vi "Periodic Tasks.vi"(8 "error in":errorcluster) -> ()   [LabVIEW 2018]
doc: "This VI runs in parallel to other tasks. It can contain as many user-defined periodic loops as you need. These can carry out PID or other sorts of timed response."
uses:
  <vilib>/Rock Robotics/WPI/Solenoid/WPI_SolenoidValue.ctl
  <vilib>/Rock Robotics/WPI/ThirdParty/Phoenix-LabVIEW/Motor Controller/Controls/CTRE_Phoenix_MotorControl_ControlMode.ctl
  <vilib>/Rock Robotics/WPI/DriverStation/WPI_DriverStationRobotMode2.ctl
  558dcaf8-7ea7-4920-b857-199f0f95a235.vi
  db2b8676-33c7-4e09-9355-13c98dcb7fd1.vi
  49744297-d732-4f26-b9df-ea13e04ead65.vi
  0c7d2dc5-c582-4743-8fb3-b9c2bdc871ef.vi
  0ab41fdd-f005-4a41-8abb-d0c1aebc8839.vi
  eb1224c5-d191-4a5a-b208-f0176ff8254b.vi
  fa0b2ed9-014b-4d02-a9e7-965de739ed34.vi
  3bc81077-0bee-49a4-9064-f6dc6ff34700.vi
  c6107473-3bbc-4d68-b130-33bb0f28684e.vi
  bc72f310-a025-467b-8a7d-9af20b832017.vi
  627df16c-e363-45ec-ab0c-cc0e3a3b33f7.vi
  9981459b-1b43-4049-8584-415fba4f8944.vi
  f90bc81b-d4ab-4cd4-9451-4feb4d491bc8.vi
  4a955322-911f-44d6-8f01-79f36aab782e.vi
  ea05d6e2-4bc2-4863-96e4-0034388c650a.vi
  93672789-ce46-4bc6-a5b5-faff44e817a8.vi
  c8be7294-c6ee-427e-ae78-3199e8744a18.vi
  1c7609ed-6cb5-470b-bbb9-41d14296924d.vi
  50b6936b-a54e-4087-a151-83919d29fb22.vi
  efed0d96-a490-4904-9cbf-ad4873da1ad9.vi
  96b11e64-b6fc-4637-b85c-b75fecbcb338.vi
  RobotStates.vi
  Robot Global Data.vi
  <vilib>/Rock Robotics/Network Tables/NT Write Number.vi
  RefNums_DriverStation.vi
  <vilib>/Rock Robotics/WPI/Utilities/WPI_GetSetVariantRefNum.vi
  RefNums_Actuators.vi
  <vilib>/Rock Robotics/WPI/Solenoid/WPI_SolenoidSetEnum.vi
  SensorReadings.vi
  Inputs_DriverStation.vi
  RefNums_Sensors.vi
  843581b2-07bb-4a5d-853d-75b7c067592b.vi
  455b4b06-4f38-49e0-865f-ae84c517b9e7.vi
panel:
  out "Sensor Loop (ms)":u32
  in  "Enable Plotting":bool
  out "Control Loop Time (ms)":u32
  out "PID Tracking":cluster{"Goal Wheel Position":dbl, dbl}(graph)={"Goal Wheel Position"=0.0, -90.17571233858979}
  out "Contribution Tracking":cluster{dbl, dbl, dbl}(graph)
  in  "N-Int":i32=50
  in  "N-Diff":i32=50
  in  "Kd":dbl=1e-06
  in  "Ki":dbl=5e-06
  in  "Kp":dbl=3e-05
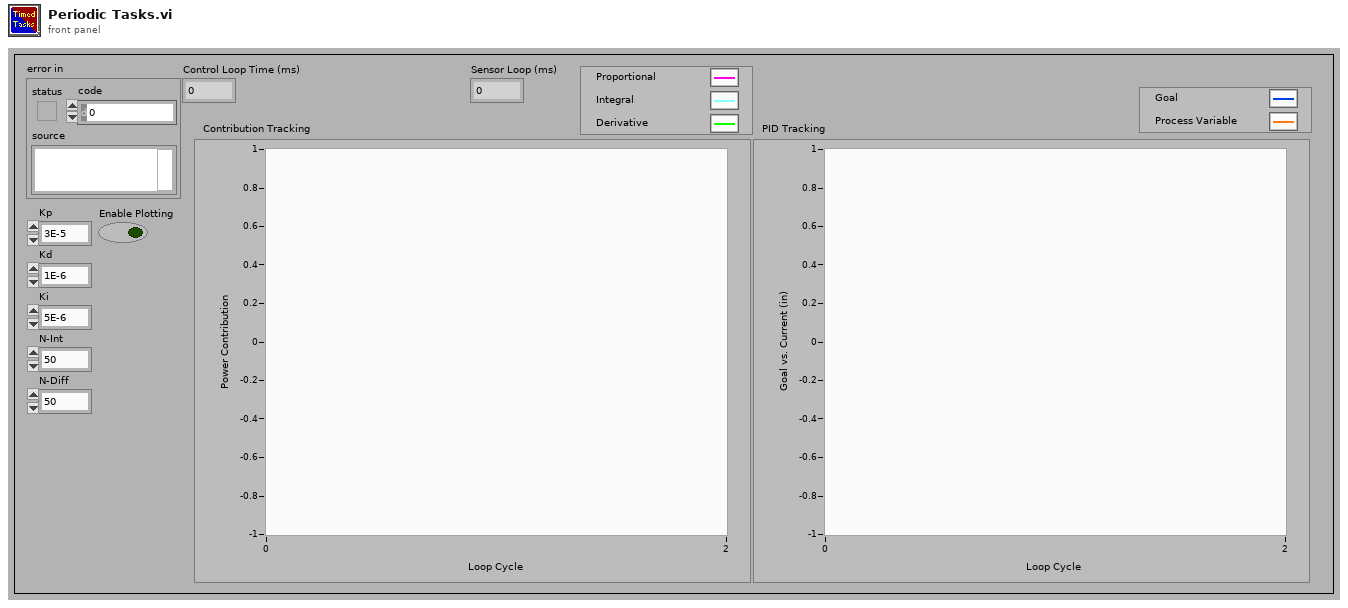
[diagram p1: front panel]
types:
  T1 = typedef "WPI_MotorControlDeviceRef.ctl" = cluster{"DeviceStatus":errorcluster, "Type":T2, "PWM":cluster{"PWM Channel":T3, "DeadBand":T4}, "CAN":cluster{"Device Number":u8, "SetOutput VI Ref":variant, "GetOutput VI Ref":variant, "Enable VI Ref":variant, "Disable VI Ref":variant, "Data":variant}, "Invert":bool, "DIO PWM":cluster{"PWM \"Enable\" Channel":T3, "DIOChannel":T5, "PWM Rate":dbl}}
  T2 = typedef "WPI_MotorControlType.ctl" = enum16{"PWM", "CAN", "DIO PWM"}
  T3 = typedef "FPGA_DIOPWMChannel.ctl" = enum8{"PWM 0", "PWM 1", "PWM 2", "PWM 3", "PWM 4", "PWM 5", "PWM 6", "PWM 7", "PWM 8", "PWM 9", "PWM MXP 0", "PWM MXP 1", "PWM MXP 2", "PWM MXP 3", "PWM MXP 4", "PWM MXP 5", "PWM MXP 6", "PWM MXP 7", "PWM MXP 8", "PWM MXP 9", "Invalid"}
  T4 = typedef "WPI_PWMDeadband.ctl" = cluster{"Name":string, "maxPositivePwm":i32, "minPositivePwm":i32, "centerPwm":i32, "maxNegativePwm":i32, "minNegativePwm":i32, "angularRange":u16}
  T5 = typedef "FPGA_DIOChannel.ctl" = enum8{"DIO 0", "DIO 1", "DIO 2", "DIO 3", "DIO 4", "DIO 5", "DIO 6", "DIO 7", "DIO 8", "DIO 9", "DIO MXP 0", "DIO MXP 1", "DIO MXP 2", "DIO MXP 3", "DIO MXP 4", "DIO MXP 5", "DIO MXP 6", "DIO MXP 7", "DIO MXP 8", "DIO MXP 9", "DIO MXP 10", "DIO MXP 11", "DIO MXP 12", "DIO MXP 13", "DIO MXP 14", "DIO MXP 15", "SPI Port CS1", "SPI Port CS2", "SPI Port CS3", "SPI Port MISO", "SPI Port MOSI", "Invalid"}
  T6 = typedef "WPI_SolenoidDevRef.ctl" = cluster{"DevStatus":errorcluster, "Pneumatics Control Module":u8, "Forward Solenoid Channel":T7, "Reverse Solenoid Channel":T7}
  T7 = typedef "WPI_SolenoidChannel.ctl" = enum8{"Solenoid 0", "Solenoid 1", "Solenoid 2", "Solenoid 3", "Solenoid 4", "Solenoid 5", "Solenoid 6", "Solenoid 7", "Invalid"}
  T8 = typedef "WPI_RobotDriveDevRef.ctl" = cluster{"DevStatus":errorcluster, "Motors[]":T1[], "Square Inputs":bool, "Max Output":dbl}
  T9 = typedef "WPI_JoystickDevRef.ctl" = cluster{"Device":T10}
  T10 = typedef "WPI_JoystickDeviceEnum.ctl" = enum16{"USB 0", "USB 1", "USB 2", "USB 3", "USB 4", "USB 5"}
  T11 = typedef "WPI_CompressorDevRef.ctl" = cluster{"DevStatus":errorcluster, "Pneumatics Control Module":u8}
  T12 = typedef "WPI_AnalogChannelDevRef.ctl" = cluster{"DevStatus":errorcluster, "Analog Channel":T13}
  T13 = typedef "FPGA_AIChannel.ctl" = enum8{"AI 0", "AI 1", "AI 2", "AI 3", "AI MXP 0", "AI MXP 1", "AI MXP 2", "AI MXP 3", "Invalid"}
  T14 = typedef "WPI_DriverStationRobotMode2.ctl" = enum16{"Autonomous Disabled", "Autonomous Enabled", "Teleop Disabled", "Teleop Enabled", "Disconnected", "Finish", "Test Disabled", "Test Enabled", "Emergency Stopped"}
  T15 = typedef "CTRE_Phoenix_MotorControl_ControlMode.ctl" = u16
  T16 = typedef "WPI_SolenoidValue.ctl" = enum16{"Off", "On", "Forward", "Reverse"}
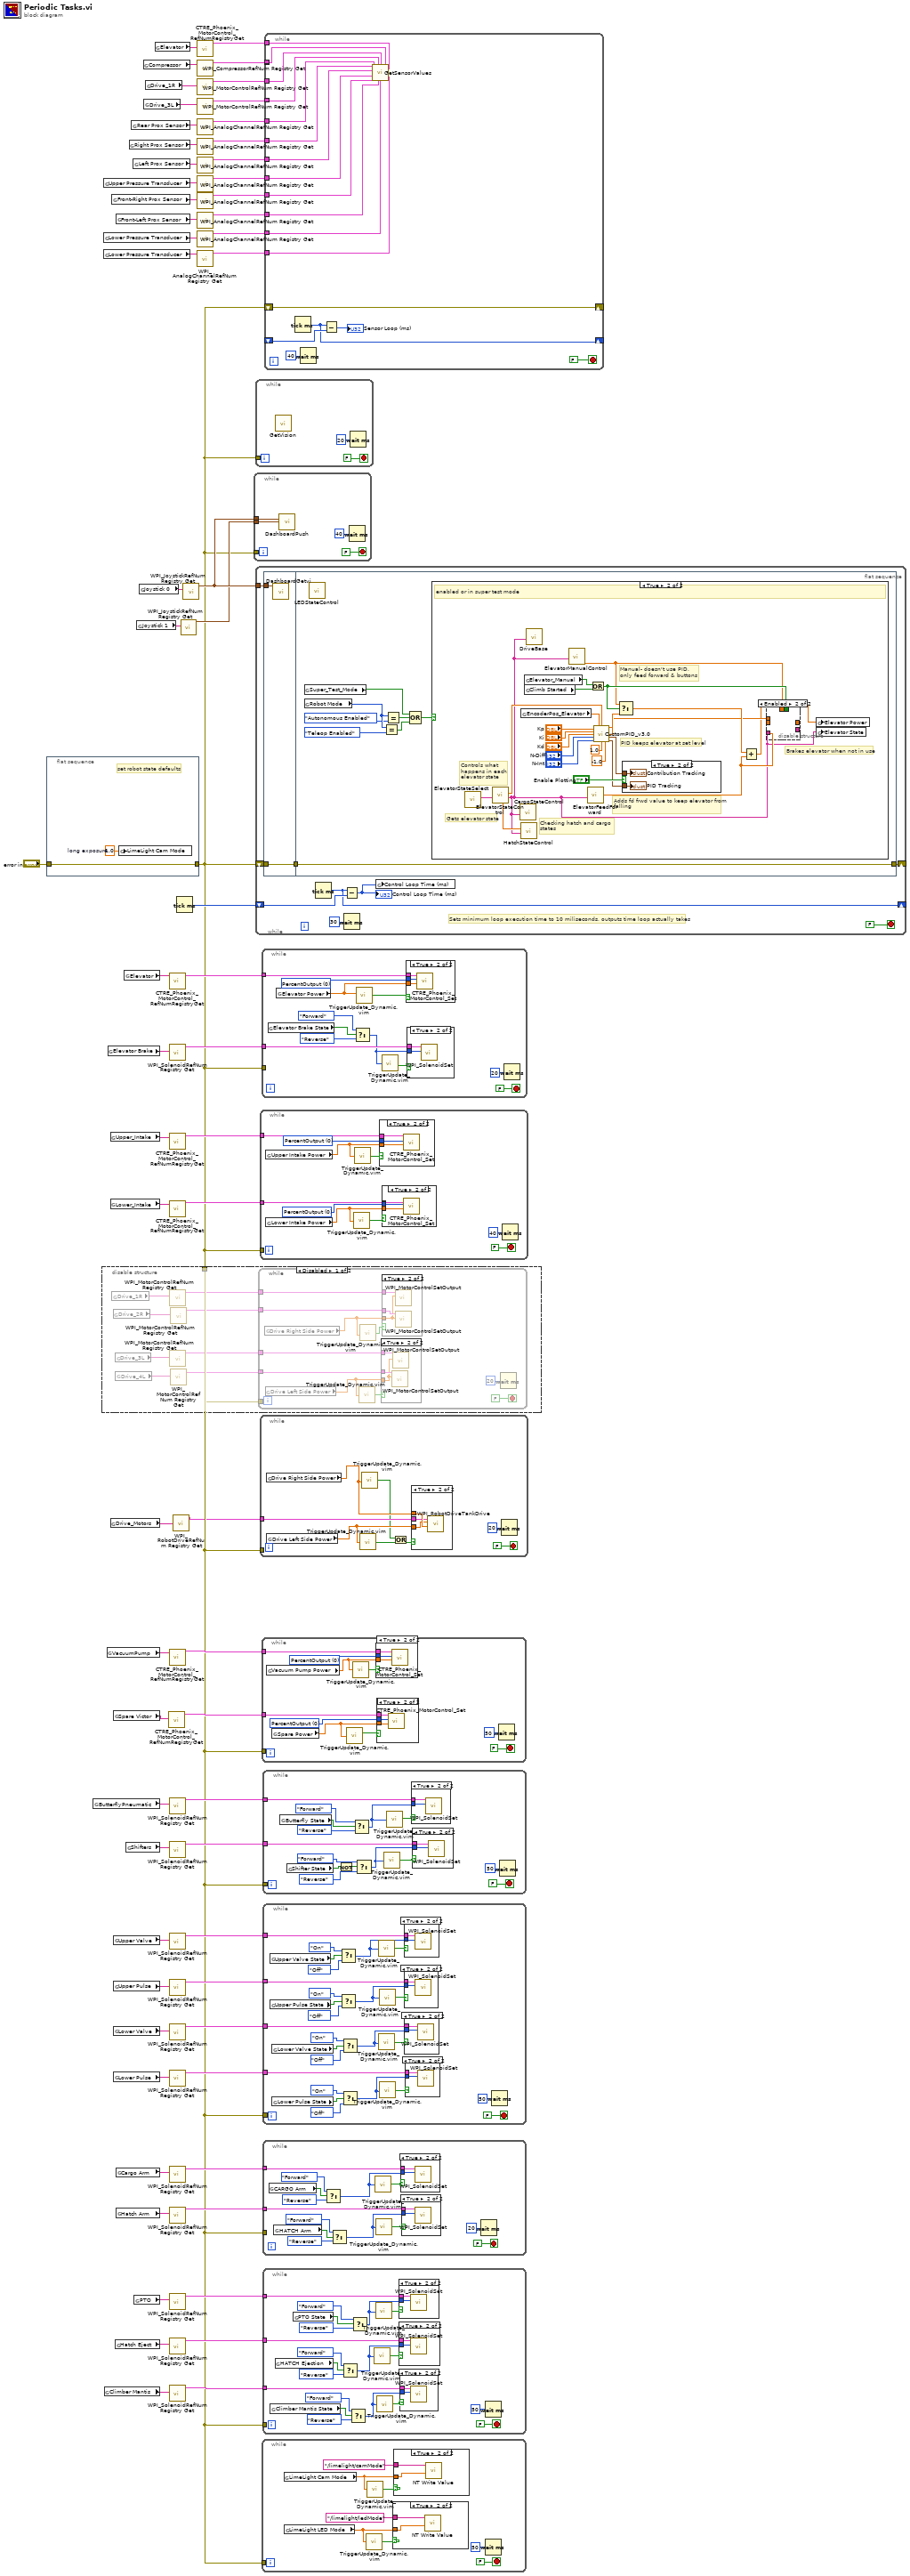
[diagram p0: block diagram]
diagram:
  n1 = flat-sequence {
    tunnel: [w69] -> w3
    tunnel: "error in" -> [w69]
    frame #0 {
      w68 = 1.0  # long exposure
      # "set robot state defaults"
      n2 = global write "RobotStates.vi" "LimeLight Cam Mode"(w68) -> ()
    }
  }
  n3 = global read "RefNums_Actuators.vi" "ButterflyPneumatic"() -> (w65:string)
  n4 = disable-structure shown="Disabled" {
    disable-tunnel: w3 -> [w70 _]
    frame Disabled {
      n5 = global read "RefNums_Actuators.vi" "Drive_1R"() -> (w72:string)
      n6 = global read "RefNums_Actuators.vi" "Drive_2R"() -> (w78:string)
      n7 = global read "RefNums_Actuators.vi" "Drive_3L"() -> (w74:string)
      n8 = global read "RefNums_Actuators.vi" "Drive_4L"() -> (w76:string)
      n9 = call <vilib>:"WPI_MotorControlRefNum Registry Get.vi"("refnum name"=w72) -> ("MotorControlDevRef"=w71:T1)  [unwired: 9 in, 1 out]
      n10 = call <vilib>:"WPI_MotorControlRefNum Registry Get.vi"("refnum name"=w74) -> ("MotorControlDevRef"=w73:T1)  [unwired: 9 in, 1 out]
      n11 = call <vilib>:"WPI_MotorControlRefNum Registry Get.vi"("refnum name"=w76) -> ("MotorControlDevRef"=w75:T1)  [unwired: 9 in, 1 out]
      n12 = call <vilib>:"WPI_MotorControlRefNum Registry Get.vi"("refnum name"=w78) -> ("MotorControlDevRef"=w77:T1)  [unwired: 9 in, 1 out]
      n13 = while {
        tunnel: w77 -> [w88]
        tunnel: w75 -> [w87]
        tunnel: w70 -> [_]
        tunnel: w73 -> [w80]
        tunnel: w71 -> [w79]
        stop <- FALSE stop-if-true
        n14 = global read "RobotStates.vi" "Drive Right Side Power"() -> (w84:dbl)
        n15 = global read "RobotStates.vi" "Drive Left Side Power"() -> (w82:dbl)
        n16 = call "TriggerUpdate_Dynamic.vim"("Trigger"=w82) -> ("Update"=w81:bool)
        n17 = call "TriggerUpdate_Dynamic.vim"("Trigger"=w84) -> ("Update"=w83:bool)
        n18 = case shown="True" w81 {
          tunnel: w87 -> [_ w91]
          tunnel: w82 -> [_ w90]
          tunnel: w80 -> [_ w89]
          frame False {
          }
          frame True {
            n19 = call <vilib>:"WPI_MotorControlSetOutput.vi"("Output"=w90, "MotorControlDevRef"=w91) -> ()  [unwired: 7 in, 3 out]
            n20 = call <vilib>:"WPI_MotorControlSetOutput.vi"("Output"=w90, "MotorControlDevRef"=w89) -> ()  [unwired: 7 in, 3 out]
          }
        }
        n21 = case shown="True" w83 {
          tunnel: w88 -> [_ w94]
          tunnel: w84 -> [_ w93]
          tunnel: w79 -> [_ w92]
          frame False {
          }
          frame True {
            n22 = call <vilib>:"WPI_MotorControlSetOutput.vi"("Output"=w93, "MotorControlDevRef"=w92) -> ()  [unwired: 7 in, 3 out]
            n23 = call <vilib>:"WPI_MotorControlSetOutput.vi"("Output"=w93, "MotorControlDevRef"=w94) -> ()  [unwired: 7 in, 3 out]
          }
        }
        n24 = Wait (ms)(milliseconds to wait=u32 20) -> ()  [unwired: 1 out]
      }
    }
    frame Enabled {
    }
  }
  n25 = global read "RefNums_Sensors.vi" "Upper Pressure Transducer"() -> (w23:string)
  n26 = global read "RefNums_Sensors.vi" "Lower Pressure Transducer"() -> (w22:string)
  n27 = global read "RefNums_Sensors.vi" "Lower Pressure Transducer"() -> (w19:string)
  n28 = global read "RefNums_Actuators.vi" "Climber Mantis"() -> (w44:string)
  n29 = global read "RefNums_Actuators.vi" "VacuumPump"() -> (w58:string)
  n30 = global read "RefNums_Actuators.vi" "Elevator Brake"() -> (w47:string)
  n31 = global read "RefNums_Actuators.vi" "Upper_Intake"() -> (w55:string)
  n32 = global read "RefNums_Actuators.vi" "Lower_Intake"() -> (w54:string)
  n33 = global read "RefNums_Actuators.vi" "Drive_Motors"() -> (w2:string)
  n34 = global read "RefNums_Sensors.vi" "Front-Right Prox Sensor"() -> (w20:string)
  n35 = global read "RefNums_Actuators.vi" "Spare Victor"() -> (w51:string)
  n36 = global read "RefNums_Actuators.vi" "Upper Valve"() -> (w40:string)
  n37 = global read "RefNums_Actuators.vi" "Upper Pulse"() -> (w61:string)
  n38 = global read "RefNums_Actuators.vi" "Lower Valve"() -> (w38:string)
  n39 = global read "RefNums_Actuators.vi" "Lower Pulse"() -> (w36:string)
  n40 = global read "RefNums_Actuators.vi" "Hatch Eject"() -> (w45:string)
  n41 = global read "RefNums_Sensors.vi" "Front-Left Prox Sensor"() -> (w21:string)
  n42 = global read "RefNums_Actuators.vi" "Cargo Arm"() -> (w57:string)
  n43 = global read "RefNums_Actuators.vi" "Hatch Arm"() -> (w46:string)
  n44 = global read "RefNums_Actuators.vi" "Elevator"() -> (w11:string)
  n45 = global read "RefNums_Actuators.vi" "Shifters"() -> (w63:string)
  n46 = global read "RefNums_Sensors.vi" "Right Prox Sensor"() -> (w27:string)
  n47 = global read "RefNums_Sensors.vi" "Rear Prox Sensor"() -> (w29:string)
  n48 = global read "RefNums_Sensors.vi" "Left Prox Sensor"() -> (w28:string)
  n49 = global read "RefNums_Actuators.vi" "PTO"() -> (w49:string)
  n50 = global read "RefNums_DriverStation.vi" "Joystick 1"() -> (w10:string)
  n51 = global read "RefNums_DriverStation.vi" "Joystick 0"() -> (w66:string)
  n52 = global read "RefNums_Actuators.vi" "Compressor"() -> (w33:string)
  n53 = global read "RefNums_Actuators.vi" "Drive_3L"() -> (w6:string)
  n54 = global read "RefNums_Actuators.vi" "Drive_1R"() -> (w7:string)
  n55 = global read "RefNums_Actuators.vi" "Elevator"() -> (w32:string)
  n56 = call <vilib>:"CTRE_Phoenix_MotorControl_RefNumRegistryGet.vi"("refnum name"=w51) -> ("PhoenixMotorControlDevRef"=w50:T1)  [unwired: 9 in, 1 out]
  n57 = call <vilib>:"CTRE_Phoenix_MotorControl_RefNumRegistryGet.vi"("refnum name"=w11) -> ("PhoenixMotorControlDevRef"=w67:T1)  [unwired: 9 in, 1 out]
  n58 = call <vilib>:"WPI_SolenoidRefNum Registry Get.vi"("refnum name"=w47) -> ("SolenoidDevRef"=w13:T6)  [unwired: 9 in, 1 out]
  n59 = call <vilib>:"CTRE_Phoenix_MotorControl_RefNumRegistryGet.vi"("refnum name"=w55) -> ("PhoenixMotorControlDevRef"=w53:T1)  [unwired: 9 in, 1 out]
  n60 = call <vilib>:"CTRE_Phoenix_MotorControl_RefNumRegistryGet.vi"("refnum name"=w54) -> ("PhoenixMotorControlDevRef"=w52:T1)  [unwired: 9 in, 1 out]
  n61 = call <vilib>:"CTRE_Phoenix_MotorControl_RefNumRegistryGet.vi"("refnum name"=w58) -> ("PhoenixMotorControlDevRef"=w59:T1)  [unwired: 9 in, 1 out]
  n62 = call <vilib>:"WPI_SolenoidRefNum Registry Get.vi"("refnum name"=w65) -> ("SolenoidDevRef"=w64:T6)  [unwired: 9 in, 1 out]
  n63 = call <vilib>:"WPI_SolenoidRefNum Registry Get.vi"("refnum name"=w63) -> ("SolenoidDevRef"=w62:T6)  [unwired: 9 in, 1 out]
  n64 = call <vilib>:"WPI_SolenoidRefNum Registry Get.vi"("refnum name"=w40) -> ("SolenoidDevRef"=w39:T6)  [unwired: 9 in, 1 out]
  n65 = call <vilib>:"WPI_SolenoidRefNum Registry Get.vi"("refnum name"=w61) -> ("SolenoidDevRef"=w60:T6)  [unwired: 9 in, 1 out]
  n66 = call <vilib>:"WPI_SolenoidRefNum Registry Get.vi"("refnum name"=w38) -> ("SolenoidDevRef"=w37:T6)  [unwired: 9 in, 1 out]
  n67 = call <vilib>:"WPI_SolenoidRefNum Registry Get.vi"("refnum name"=w36) -> ("SolenoidDevRef"=w35:T6)  [unwired: 9 in, 1 out]
  n68 = call <vilib>:"WPI_SolenoidRefNum Registry Get.vi"("refnum name"=w57) -> ("SolenoidDevRef"=w56:T6)  [unwired: 9 in, 1 out]
  n69 = call <vilib>:"WPI_SolenoidRefNum Registry Get.vi"("refnum name"=w46) -> ("SolenoidDevRef"=w43:T6)  [unwired: 9 in, 1 out]
  n70 = call <vilib>:"WPI_SolenoidRefNum Registry Get.vi"("refnum name"=w49) -> ("SolenoidDevRef"=w48:T6)  [unwired: 9 in, 1 out]
  n71 = call <vilib>:"WPI_SolenoidRefNum Registry Get.vi"("refnum name"=w45) -> ("SolenoidDevRef"=w42:T6)  [unwired: 9 in, 1 out]
  n72 = call <vilib>:"WPI_SolenoidRefNum Registry Get.vi"("refnum name"=w44) -> ("SolenoidDevRef"=w41:T6)  [unwired: 9 in, 1 out]
  n73 = call <vilib>:"WPI_RobotDriveRefNum Registry Get.vi"("refnum name"=w2) -> ("RobotDriveDevRef"=w1:T8)  [unwired: 9 in, 1 out]
  n74 = Tick Count (ms)() -> (millisecond timer value=w34:u32)
  n75 = call <vilib>:"WPI_JoystickRefNum Registry Get.vi"("refnum name"=w10) -> ("JoystickDevRef"=w9:T9)  [unwired: 9 in, 1 out]
  n76 = call <vilib>:"WPI_JoystickRefNum Registry Get.vi"("refnum name"=w66) -> ("JoystickDevRef"=w12:T9)  [unwired: 9 in, 1 out]
  n77 = call <vilib>:"CTRE_Phoenix_MotorControl_RefNumRegistryGet.vi"("refnum name"=w32) -> ("PhoenixMotorControlDevRef"=w31:T1)  [unwired: 9 in, 1 out]
  n78 = call <vilib>:"WPI_CompressorRefNum Registry Get.vi"("refnum name"=w33) -> ("CompressorDevRef"=w30:T11)  [unwired: 9 in, 1 out]
  n79 = call <vilib>:"WPI_MotorControlRefNum Registry Get.vi"("refnum name"=w7) -> ("MotorControlDevRef"=w5:T1)  [unwired: 9 in, 1 out]
  n80 = call <vilib>:"WPI_MotorControlRefNum Registry Get.vi"("refnum name"=w6) -> ("MotorControlDevRef"=w4:T1)  [unwired: 9 in, 1 out]
  n81 = call <vilib>:"WPI_AnalogChannelRefNum Registry Get.vi"("refnum name"=w29) -> ("AIDeviceRef"=w26:T12)  [unwired: 9 in, 1 out]
  n82 = call <vilib>:"WPI_AnalogChannelRefNum Registry Get.vi"("refnum name"=w27) -> ("AIDeviceRef"=w25:T12)  [unwired: 9 in, 1 out]
  n83 = call <vilib>:"WPI_AnalogChannelRefNum Registry Get.vi"("refnum name"=w28) -> ("AIDeviceRef"=w24:T12)  [unwired: 9 in, 1 out]
  n84 = call <vilib>:"WPI_AnalogChannelRefNum Registry Get.vi"("refnum name"=w23) -> ("AIDeviceRef"=w18:T12)  [unwired: 9 in, 1 out]
  n85 = call <vilib>:"WPI_AnalogChannelRefNum Registry Get.vi"("refnum name"=w20) -> ("AIDeviceRef"=w17:T12)  [unwired: 9 in, 1 out]
  n86 = call <vilib>:"WPI_AnalogChannelRefNum Registry Get.vi"("refnum name"=w21) -> ("AIDeviceRef"=w16:T12)  [unwired: 9 in, 1 out]
  n87 = call <vilib>:"WPI_AnalogChannelRefNum Registry Get.vi"("refnum name"=w22) -> ("AIDeviceRef"=w15:T12)  [unwired: 9 in, 1 out]
  n88 = call <vilib>:"WPI_AnalogChannelRefNum Registry Get.vi"("refnum name"=w19) -> ("AIDeviceRef"=w14:T12)  [unwired: 9 in, 1 out]
  n89 = while {
    tunnel: w12 -> [w97]
    tunnel: w3 -> [_]
    tunnel: w9 -> [w95]
    stop <- FALSE stop-if-true
    n90 = call "DashboardPush.vi"("Joystick 0 Ref"=w97, "Joystick 1 Ref"=w95) -> ()  [unwired: 14 in]
    n91 = Wait (ms)(milliseconds to wait=u32 40) -> ()  [unwired: 1 out]
  }
  n92 = while {
    tunnel: w3 -> [_]
    stop <- FALSE stop-if-true
    n93 = call "GetVision.vi"() -> ()  [unwired: 12 in]
    n94 = Wait (ms)(milliseconds to wait=u32 20) -> ()  [unwired: 1 out]
  }
  n95 = while {
    shift-right: [w105] -> _
    shift-left: w3 -> [w107]
    tunnel: w12 -> [w104]
    shift-right: [w102] -> _
    shift-left: w34 -> [w103]
    stop <- FALSE stop-if-true
    # "Sets minimum loop execution time to 10 miliseconds, outputs time loop actually takes"
    n96 = flat-sequence {
      tunnel: w104 -> [w111]
      tunnel: w107 -> [w110]
      tunnel: [w110] -> w106
      tunnel: w106 -> [w119]
      tunnel: [w119] -> w105
      frame #0 {
        n97 = call "DashboardGetvi.vi"("Joystick 1"=w111) -> ()  [unwired: 9 in]
      }
      frame #1 {
        n98 = global read "Inputs_DriverStation.vi" "Super_Test_Mode"() -> (w112:bool)
        n99 = global read "Robot Global Data.vi" "Robot Mode"() -> (w116:T14)
        n100 = call "LEDStateControl.vi"() -> ()  [unwired: 12 in]
        n101 = Equal?(x=w116, y=WPI_DriverStationRobotMode2."Teleop Enabled") -> (x = y?=w117:bool)
        n102 = Equal?(x=w116, y=WPI_DriverStationRobotMode2."Autonomous Enabled") -> (x = y?=w118:bool)
        n103 = Compound Arithmetic op=OR(w112, w118, w117) -> (w113:bool)
        n104 = case shown="True" w113 {
          frame False {
            # "disabled and not in super test mode"
          }
          frame True {
            # "Brakes elevator when not in use"
            # "PID keeps elevator at set level"
            # "Manual- doesn't use PID,\nonly feed forward & buttons"
            # "Adds fd frwd value to keep elevator from falling"
            # "Checking hatch and cargo \nstates"
            # "Controls what\nhappens in each \nelevator state"
            # "Gets elevator state"
            # "enabled or in super test mode"
            n105 = call "ElevatorStateSelect.vi"() -> ("Elevator State"=w140:string)  [unwired: 11 in]
            n106 = call "ElevatorStateControl.vi"("Elevator State"=w140) -> ("Elevator State Out"=w121:string, "Target Elevator Position"=w138:dbl, "Target Vacuum Pump Power"=w127:dbl)  [unwired: 8 in]
            n107 = call "CargoStateControl.vi"("Elevator State"=w121) -> ()  [unwired: 11 in]
            n108 = call "HatchStateControl.vi"("Elevator State"=w121, "Vacuum Pump Power"=w127) -> ()  [unwired: 10 in]
            n109 = global read "SensorReadings.vi" "EncoderPos_Elevator"() -> (w137:dbl)
            n110 = global read "Inputs_DriverStation.vi" "Elevator_Manual"() -> (w123:bool)
            n111 = global read "RobotStates.vi" "Climb Started"() -> (w122:bool)
            n112 = call "DriveBase.vi"("Elevator State"=w121) -> ()  [unwired: 11 in]
            n113 = call "ElevatorManualControl.vi"("Elevator State"=w121) -> ("Manual Contribution"=w126:dbl)  [unwired: 10 in]
            n114 = call "ElevatorFeedForward.vi"("Elevator State"=w121) -> ("Feed Forward Contribution"=w124:dbl)  [unwired: 10 in]
            n115 = Or(x=w123, y=w122) -> (x .or. y?=w143:bool)
            n116 = call "CustomPID_v3.0.vi"("Kp"="Kp", "Process Variable"=w137, "Goal"=w138, "Ki"="Ki", "Kd"="Kd", "N-Diff"="N-Diff", "N-Int"="N-Int", "Max Ouput"=1.0, "Min Output"=-1.0) -> ("Current Error"=w125:dbl, "Command"=w139:dbl, "Contribution Tracking"=w129:cluster{dbl, dbl, dbl}, "PID Tracking"=w128:cluster{"Goal Wheel Position":dbl, dbl})  [unwired: 3 in]
            n117 = Select(t=w126, s=w143, f=w139) -> (s? t:f=w141:dbl)
            n118 = case shown="True" "Enable Plotting" {
              tunnel: w129 -> [_ w153]
              tunnel: w128 -> [_ w152]
              frame False {
              }
              frame True {
                "Contribution Tracking" <- w153
                "PID Tracking" <- w152
              }
            }
            n119 = Add(x=w141, y=w124) -> (x+y=w120:dbl)
            n120 = disable-structure shown="Enabled" {
              disable-tunnel: w143 -> [w151 _]
              disable-tunnel: _ -> [w150 _]
              disable-tunnel: [w149 _] -> _
              disable-tunnel: [w148 _] -> _
              disable-tunnel: w126 -> [w147 _]
              disable-tunnel: w125 -> [w146 _]
              disable-tunnel: w124 -> [w145 _]
              disable-tunnel: w121 -> [w144 _]
              frame Disabled {
                n121 = call "ElevatorBrake.vi"("Elevator Manual Mode"=w151, "Manual Movement"=w147, "Feed Forward Contribution"=w145, "Elevator State In"=w144, "Elevator Power In"=w150, "Elevator Error"=w146) -> ("Elevator State Out"=w148:string, "Elevator Power Out"=w149:dbl)  [unwired: 4 in]
              }
              frame Enabled {
              }
            }
            n122 = global write "RobotStates.vi" "Elevator Power"(w120) -> ()
            n123 = global write "RobotStates.vi" "Elevator State"(w121) -> ()
          }
        }
      }
    }
    n124 = Tick Count (ms)() -> (millisecond timer value=w102:u32)
    n125 = Wait (ms)(milliseconds to wait=u32 30) -> ()  [unwired: 1 out]
    n126 = Subtract(x=w102, y=w103) -> (x-y=w101:u32)
    "Control Loop Time (ms)" <- w101
    n127 = global write "SensorReadings.vi" "Control Loop Time (ms)"(w101) -> ()
  }
  n128 = while {
    tunnel: w53 -> [w163]
    tunnel: w52 -> [w162]
    tunnel: w3 -> [_]
    stop <- FALSE stop-if-true
    w160 = T15 0 items=["PercentOutput"=0, "Position"=1, "Velocity"=2, "Current"=3, "Follower"=5, "MotionProfile"=6, "MotionMagic"=7, "MotionProfileArc"=10, "Disabled"=15] ("Control Mode")
    w161 = T15 0 items=["PercentOutput"=0, "Position"=1, "Velocity"=2, "Current"=3, "Follower"=5, "MotionProfile"=6, "MotionMagic"=7, "MotionProfileArc"=10, "Disabled"=15] ("Control Mode")
    n129 = global read "RobotStates.vi" "Upper Intake Power"() -> (w157:dbl)
    n130 = global read "RobotStates.vi" "Lower Intake Power"() -> (w155:dbl)
    n131 = call "TriggerUpdate_Dynamic.vim"("Trigger"=w155) -> ("Update"=w154:bool)
    n132 = call "TriggerUpdate_Dynamic.vim"("Trigger"=w157) -> ("Update"=w156:bool)
    n133 = case shown="True" w156 {
      tunnel: w163 -> [_ w169]
      tunnel: w161 -> [_ w168]
      tunnel: w157 -> [_ w167]
      frame False {
      }
      frame True {
        n134 = call <vilib>:"CTRE_Phoenix_MotorControl_Set.vi"("Output"=w167, "Control Mode"=w168, "PhoenixMotorControlDevRef"=w169) -> ()  [unwired: 7 in, 2 out]
      }
    }
    n135 = case shown="True" w154 {
      tunnel: w162 -> [_ w166]
      tunnel: w160 -> [_ w165]
      tunnel: w155 -> [_ w164]
      frame False {
      }
      frame True {
        n136 = call <vilib>:"CTRE_Phoenix_MotorControl_Set.vi"("Output"=w164, "Control Mode"=w165, "PhoenixMotorControlDevRef"=w166) -> ()  [unwired: 7 in, 2 out]
      }
    }
    n137 = Wait (ms)(milliseconds to wait=u32 40) -> ()  [unwired: 1 out]
  }
  n138 = while {
    tunnel: w1 -> [w177]
    tunnel: w3 -> [_]
    stop <- FALSE stop-if-true
    n139 = global read "RobotStates.vi" "Drive Right Side Power"() -> (w172:dbl)
    n140 = global read "RobotStates.vi" "Drive Left Side Power"() -> (w174:dbl)
    n141 = call "TriggerUpdate_Dynamic.vim"("Trigger"=w174) -> ("Update"=w173:bool)
    n142 = call "TriggerUpdate_Dynamic.vim"("Trigger"=w172) -> ("Update"=w170:bool)
    n143 = Or(x=w170, y=w173) -> (x .or. y?=w171:bool)
    n144 = case shown="True" w171 {
      tunnel: w177 -> [_ w178]
      tunnel: w174 -> [_ w179]
      tunnel: w172 -> [_ w180]
      frame False {
      }
      frame True {
        n145 = call <vilib>:"WPI_RobotDriveTankDrive.vi"("Right axis value"=w180, "Left axis value"=w179, "RobotDriveDevRef"=w178) -> ()  [unwired: 6 in, 3 out]
      }
    }
    n146 = Wait (ms)(milliseconds to wait=u32 20) -> ()  [unwired: 1 out]
  }
  n147 = while {
    tunnel: w3 -> [_]
    tunnel: w13 -> [w187]
    tunnel: w67 -> [w186]
    stop <- FALSE stop-if-true
    w185 = T15 0 items=["PercentOutput"=0, "Position"=1, "Velocity"=2, "Current"=3, "Follower"=5, "MotionProfile"=6, "MotionMagic"=7, "MotionProfileArc"=10, "Disabled"=15] ("Control Mode")
    n148 = global read "RobotStates.vi" "Elevator Brake State"() -> (w190:bool)
    n149 = global read "RobotStates.vi" "Elevator Power"() -> (w184:dbl)
    n150 = Select(t=WPI_SolenoidValue."Forward" ("Value"), s=w190, f=WPI_SolenoidValue."Reverse") -> (s? t:f=w182:T16)
    n151 = call "TriggerUpdate_Dynamic.vim"("Trigger"=w184) -> ("Update"=w183:bool)
    n152 = call "TriggerUpdate_Dynamic.vim"("Trigger"=w182) -> ("Update"=w181:bool)
    n153 = case shown="True" w183 {
      tunnel: w186 -> [_ w195]
      tunnel: w185 -> [_ w194]
      tunnel: w184 -> [_ w193]
      frame False {
      }
      frame True {
        n154 = call <vilib>:"CTRE_Phoenix_MotorControl_Set.vi"("Output"=w193, "Control Mode"=w194, "PhoenixMotorControlDevRef"=w195) -> ()  [unwired: 7 in, 2 out]
      }
    }
    n155 = case shown="True" w181 {
      tunnel: w187 -> [_ w197]
      tunnel: w182 -> [_ w196]
      frame False {
      }
      frame True {
        n156 = call-poly <vilib>:"WPI_SolenoidSet.vi"("Value"=w196, "SolenoidDevRef"=w197) -> ()  [unwired: 8 in, 2 out]
      }
    }
    n157 = Wait (ms)(milliseconds to wait=u32 20) -> ()  [unwired: 1 out]
  }
  n158 = while {
    tunnel: w59 -> [w207]
    tunnel: w50 -> [w206]
    tunnel: w3 -> [_]
    stop <- FALSE stop-if-true
    w198 = T15 0 items=["PercentOutput"=0, "Position"=1, "Velocity"=2, "Current"=3, "Follower"=5, "MotionProfile"=6, "MotionMagic"=7, "MotionProfileArc"=10, "Disabled"=15] ("Control Mode")
    w205 = T15 0 items=["PercentOutput"=0, "Position"=1, "Velocity"=2, "Current"=3, "Follower"=5, "MotionProfile"=6, "MotionMagic"=7, "MotionProfileArc"=10, "Disabled"=15] ("Control Mode")
    n159 = global read "RobotStates.vi" "Vacuum Pump Power"() -> (w202:dbl)
    n160 = global read "RobotStates.vi" "Spare Power"() -> (w200:dbl)
    n161 = call "TriggerUpdate_Dynamic.vim"("Trigger"=w200) -> ("Update"=w199:bool)
    n162 = call "TriggerUpdate_Dynamic.vim"("Trigger"=w202) -> ("Update"=w201:bool)
    n163 = case shown="True" w201 {
      tunnel: w207 -> [_ w213]
      tunnel: w205 -> [_ w212]
      tunnel: w202 -> [_ w211]
      frame False {
      }
      frame True {
        n164 = call <vilib>:"CTRE_Phoenix_MotorControl_Set.vi"("Output"=w211, "Control Mode"=w212, "PhoenixMotorControlDevRef"=w213) -> ()  [unwired: 7 in, 2 out]
      }
    }
    n165 = case shown="True" w199 {
      tunnel: w206 -> [_ w210]
      tunnel: w198 -> [_ w209]
      tunnel: w200 -> [_ w208]
      frame False {
      }
      frame True {
        n166 = call <vilib>:"CTRE_Phoenix_MotorControl_Set.vi"("Output"=w208, "Control Mode"=w209, "PhoenixMotorControlDevRef"=w210) -> ()  [unwired: 7 in, 2 out]
      }
    }
    n167 = Wait (ms)(milliseconds to wait=u32 50) -> ()  [unwired: 1 out]
  }
  n168 = while {
    tunnel: w3 -> [_]
    stop <- FALSE stop-if-true
    n169 = global read "RobotStates.vi" "LimeLight Cam Mode"() -> (w214:dbl)
    n170 = global read "RobotStates.vi" "LimeLight LED Mode"() -> (w217:dbl)
    n171 = call "TriggerUpdate_Dynamic.vim"("Trigger"=w217) -> ("Update"=w219:bool)
    n172 = call "TriggerUpdate_Dynamic.vim"("Trigger"=w214) -> ("Update"=w216:bool)
    n173 = case shown="True" w219 {
      tunnel: "/limelight/ledMode" ("Name") -> [_ w225]
      tunnel: w217 -> [_ w224]
      frame False {
      }
      frame True {
        n174 = call-poly <vilib>:"NT Write Value.vi"("Numeric"=w224, "Name"=w225) -> ()  [unwired: 9 in, 1 out]
      }
    }
    n175 = case shown="True" w216 {
      tunnel: "/limelight/camMode" ("Name") -> [_ w223]
      tunnel: w214 -> [_ w222]
      frame False {
      }
      frame True {
        n176 = call-poly <vilib>:"NT Write Value.vi"("Numeric"=w222, "Name"=w223) -> ()  [unwired: 9 in, 1 out]
      }
    }
    n177 = Wait (ms)(milliseconds to wait=u32 50) -> ()  [unwired: 1 out]
  }
  n178 = while {
    tunnel: w56 -> [w239]
    tunnel: w43 -> [w238]
    tunnel: w3 -> [_]
    stop <- FALSE stop-if-true
    n179 = global read "RobotStates.vi" "CARGO Arm"() -> (w237:bool)
    n180 = global read "RobotStates.vi" "HATCH Arm"() -> (w234:bool)
    n181 = Select(t=WPI_SolenoidValue."Forward" ("Value"), s=w237, f=WPI_SolenoidValue."Reverse") -> (s? t:f=w229:T16)
    n182 = Select(t=WPI_SolenoidValue."Forward" ("Value"), s=w234, f=WPI_SolenoidValue."Reverse") -> (s? t:f=w227:T16)
    n183 = call "TriggerUpdate_Dynamic.vim"("Trigger"=w229) -> ("Update"=w228:bool)
    n184 = call "TriggerUpdate_Dynamic.vim"("Trigger"=w227) -> ("Update"=w226:bool)
    n185 = case shown="True" w228 {
      tunnel: w239 -> [_ w243]
      tunnel: w229 -> [_ w242]
      frame False {
      }
      frame True {
        n186 = call-poly <vilib>:"WPI_SolenoidSet.vi"("Value"=w242, "SolenoidDevRef"=w243) -> ()  [unwired: 8 in, 2 out]
      }
    }
    n187 = case shown="True" w226 {
      tunnel: w238 -> [_ w241]
      tunnel: w227 -> [_ w240]
      frame False {
      }
      frame True {
        n188 = call-poly <vilib>:"WPI_SolenoidSet.vi"("Value"=w240, "SolenoidDevRef"=w241) -> ()  [unwired: 8 in, 2 out]
      }
    }
    n189 = Wait (ms)(milliseconds to wait=u32 20) -> ()  [unwired: 1 out]
  }
  n190 = while {
    tunnel: w48 -> [w263]
    tunnel: w42 -> [w262]
    tunnel: w41 -> [w261]
    tunnel: w3 -> [_]
    stop <- FALSE stop-if-true
    n191 = global read "RobotStates.vi" "Climber Mantis State"() -> (w256:bool)
    n192 = global read "RobotStates.vi" "HATCH Ejection"() -> (w258:bool)
    n193 = global read "RobotStates.vi" "PTO State"() -> (w244:bool)
    n194 = Select(t=WPI_SolenoidValue."Forward" ("Value"), s=w258, f=WPI_SolenoidValue."Reverse") -> (s? t:f=w248:T16)
    n195 = Select(t=WPI_SolenoidValue."Forward" ("Value"), s=w256, f=WPI_SolenoidValue."Reverse") -> (s? t:f=w246:T16)
    n196 = Select(t=WPI_SolenoidValue."Forward" ("Value"), s=w244, f=WPI_SolenoidValue."Reverse") -> (s? t:f=w250:T16)
    n197 = call "TriggerUpdate_Dynamic.vim"("Trigger"=w248) -> ("Update"=w247:bool)
    n198 = call "TriggerUpdate_Dynamic.vim"("Trigger"=w250) -> ("Update"=w249:bool)
    n199 = call "TriggerUpdate_Dynamic.vim"("Trigger"=w246) -> ("Update"=w245:bool)
    n200 = case shown="True" w249 {
      tunnel: w263 -> [_ w269]
      tunnel: w250 -> [_ w268]
      frame False {
      }
      frame True {
        n201 = call-poly <vilib>:"WPI_SolenoidSet.vi"("Value"=w268, "SolenoidDevRef"=w269) -> ()  [unwired: 8 in, 2 out]
      }
    }
    n202 = case shown="True" w247 {
      tunnel: w262 -> [_ w267]
      tunnel: w248 -> [_ w266]
      frame False {
      }
      frame True {
        n203 = call-poly <vilib>:"WPI_SolenoidSet.vi"("Value"=w266, "SolenoidDevRef"=w267) -> ()  [unwired: 8 in, 2 out]
      }
    }
    n204 = case shown="True" w245 {
      tunnel: w261 -> [_ w265]
      tunnel: w246 -> [_ w264]
      frame False {
      }
      frame True {
        n205 = call-poly <vilib>:"WPI_SolenoidSet.vi"("Value"=w264, "SolenoidDevRef"=w265) -> ()  [unwired: 8 in, 2 out]
      }
    }
    n206 = Wait (ms)(milliseconds to wait=u32 50) -> ()  [unwired: 1 out]
  }
  n207 = while {
    tunnel: w64 -> [w284]
    tunnel: w62 -> [w283]
    tunnel: w3 -> [_]
    stop <- FALSE stop-if-true
    n208 = global read "RobotStates.vi" "Butterfly State"() -> (w280:bool)
    n209 = global read "RobotStates.vi" "Shifter State"() -> (w279:bool)
    n210 = Not(x=w279) -> (.not. x?=w270:bool)
    n211 = Select(t=WPI_SolenoidValue."Forward" ("Value"), s=w280, f=WPI_SolenoidValue."Reverse") -> (s? t:f=w274:T16)
    n212 = Select(t=WPI_SolenoidValue."Forward" ("Value"), s=w270, f=WPI_SolenoidValue."Reverse") -> (s? t:f=w272:T16)
    n213 = call "TriggerUpdate_Dynamic.vim"("Trigger"=w272) -> ("Update"=w271:bool)
    n214 = call "TriggerUpdate_Dynamic.vim"("Trigger"=w274) -> ("Update"=w273:bool)
    n215 = case shown="True" w273 {
      tunnel: w284 -> [_ w288]
      tunnel: w274 -> [_ w287]
      frame False {
      }
      frame True {
        n216 = call-poly <vilib>:"WPI_SolenoidSet.vi"("Value"=w287, "SolenoidDevRef"=w288) -> ()  [unwired: 8 in, 2 out]
      }
    }
    n217 = case shown="True" w271 {
      tunnel: w283 -> [_ w286]
      tunnel: w272 -> [_ w285]
      frame False {
      }
      frame True {
        n218 = call-poly <vilib>:"WPI_SolenoidSet.vi"("Value"=w285, "SolenoidDevRef"=w286) -> ()  [unwired: 8 in, 2 out]
      }
    }
    n219 = Wait (ms)(milliseconds to wait=u32 50) -> ()  [unwired: 1 out]
  }
  n220 = while {
    tunnel: w60 -> [w314]
    tunnel: w39 -> [w313]
    tunnel: w37 -> [w312]
    tunnel: w35 -> [w311]
    tunnel: w3 -> [_]
    stop <- FALSE stop-if-true
    n221 = global read "RobotStates.vi" "Upper Valve State"() -> (w307:bool)
    n222 = global read "RobotStates.vi" "Upper Pulse State"() -> (w310:bool)
    n223 = global read "RobotStates.vi" "Lower Valve State"() -> (w304:bool)
    n224 = global read "RobotStates.vi" "Lower Pulse State"() -> (w301:bool)
    n225 = Select(t=WPI_SolenoidValue."On" ("Value"), s=w307, f=WPI_SolenoidValue."Off") -> (s? t:f=w296:T16)
    n226 = Select(t=WPI_SolenoidValue."On" ("Value"), s=w310, f=WPI_SolenoidValue."Off") -> (s? t:f=w294:T16)
    n227 = Select(t=WPI_SolenoidValue."On" ("Value"), s=w304, f=WPI_SolenoidValue."Off") -> (s? t:f=w292:T16)
    n228 = Select(t=WPI_SolenoidValue."On" ("Value"), s=w301, f=WPI_SolenoidValue."Off") -> (s? t:f=w290:T16)
    n229 = call "TriggerUpdate_Dynamic.vim"("Trigger"=w296) -> ("Update"=w295:bool)
    n230 = call "TriggerUpdate_Dynamic.vim"("Trigger"=w292) -> ("Update"=w291:bool)
    n231 = call "TriggerUpdate_Dynamic.vim"("Trigger"=w290) -> ("Update"=w289:bool)
    n232 = call "TriggerUpdate_Dynamic.vim"("Trigger"=w294) -> ("Update"=w293:bool)
    n233 = case shown="True" w295 {
      tunnel: w313 -> [_ w322]
      tunnel: w296 -> [_ w321]
      frame False {
      }
      frame True {
        n234 = call-poly <vilib>:"WPI_SolenoidSet.vi"("Value"=w321, "SolenoidDevRef"=w322) -> ()  [unwired: 8 in, 2 out]
      }
    }
    n235 = case shown="True" w293 {
      tunnel: w314 -> [_ w320]
      tunnel: w294 -> [_ w319]
      frame False {
      }
      frame True {
        n236 = call-poly <vilib>:"WPI_SolenoidSet.vi"("Value"=w319, "SolenoidDevRef"=w320) -> ()  [unwired: 8 in, 2 out]
      }
    }
    n237 = case shown="True" w291 {
      tunnel: w312 -> [_ w318]
      tunnel: w292 -> [_ w317]
      frame False {
      }
      frame True {
        n238 = call-poly <vilib>:"WPI_SolenoidSet.vi"("Value"=w317, "SolenoidDevRef"=w318) -> ()  [unwired: 8 in, 2 out]
      }
    }
    n239 = case shown="True" w289 {
      tunnel: w311 -> [_ w316]
      tunnel: w290 -> [_ w315]
      frame False {
      }
      frame True {
        n240 = call-poly <vilib>:"WPI_SolenoidSet.vi"("Value"=w315, "SolenoidDevRef"=w316) -> ()  [unwired: 8 in, 2 out]
      }
    }
    n241 = Wait (ms)(milliseconds to wait=u32 50) -> ()  [unwired: 1 out]
  }
  n242 = while {
    shift-right: [w338] -> _
    shift-left: w3 -> [w338]
    shift-right: [w335] -> _
    shift-left: _ -> [w336]
    tunnel: w31 -> [w334]
    tunnel: [w323] -> _
    tunnel: w30 -> [w323]
    tunnel: w5 -> [w333]
    tunnel: w4 -> [w332]
    tunnel: w26 -> [w331]
    tunnel: w25 -> [w330]
    tunnel: w24 -> [w329]
    tunnel: w18 -> [w328]
    tunnel: w17 -> [w327]
    tunnel: w16 -> [w326]
    tunnel: w15 -> [w325]
    tunnel: w14 -> [w324]
    stop <- FALSE stop-if-true
    n243 = Tick Count (ms)() -> (millisecond timer value=w335:u32)
    n244 = Wait (ms)(milliseconds to wait=u32 40) -> ()  [unwired: 1 out]
    n245 = Subtract(x=w335, y=w336) -> (x-y=→"Sensor Loop (ms)":u32)
    n246 = call "GetSensorValues.vi"("Ref_LeftDriveEncoder"=w333, "Ref_RightDriveEncoder"=w332, "Rear Prox Sensor"=w331, "Right Prox Sensor"=w330, "Left Prox Sensor"=w329, "Upper Pressure Transducer"=w328, "Ref_Compressor"=w323, "Front-Right Prox Sensor"=w327, "Ref_ElevatorEncoder"=w334, "Front-Left Prox Sensor"=w326, "Lower Pressure Transducer"=w325, "Tank Pressure Transducer"=w324) -> ()  [unwired: 16 in]
  }
